vi "CIPC_String_Tag.vi"() -> (3 "CIF_CIPC_Chn_Double.lvclass":refnum<class "CIF_CIPC_Chn_String.lvclass">)   [LabVIEW 2021, in "CIF_CIPC_Chn_String.lvclass"]
uses:
  CIF_CIPC_Chn_String.lvclass
  CIF_CIPC_Chn_String.lvclass/CIF_CIPC_Chn_String.ctl
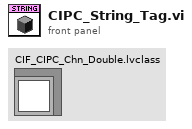
[diagram p1: front panel]
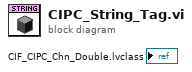
[diagram p0: block diagram]
diagram:
